vi "DigitalIOWrapper.vi"(0 "error in":errorcluster, 2 "Component IDs":T1[](array[typedef]), 3 "True Only (T)":bool=TRUE) -> (1 "error out":errorcluster, 4 "Changed_IO":T2(array[cluster]))   [LabVIEW 2015]
doc: "Fill the Component IDs array with the full names of digital inputs of interest. Returns the name and digital IO state of any input that has changed since last time.\n\nIf True Only is set, then only returns inputs whose value has changed to true (state != 0)"
uses:
  ROS/Code/SubVIs/DigitalIOComponents.ctl
panel:
  out "changed_io size":i32
  in  "EventWrappers":T2(array[cluster])
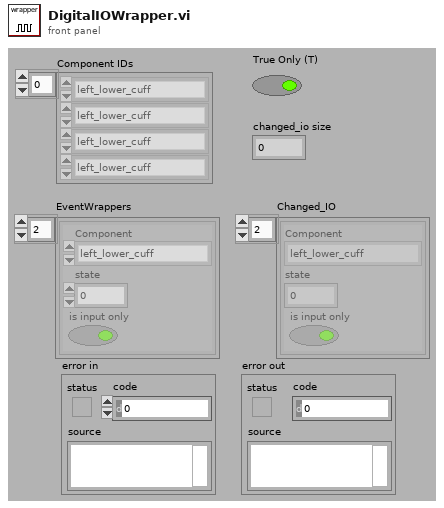
[diagram p1: front panel]
types:
  T1 = typedef "DigitalIOComponents.ctl" = enum16{"left_lower_cuff", "right_lower_cuff", "left_lower_button", "right_lower_button", "left_upper_button", "right_upper_button", "left_shoulder_button", "right_shoulder_button"}
  T2 = cluster{"Component":T1, "state":i8, "is input only":bool}[]
  T3 = cluster{"Component":T1, "state":i8, "is input only":bool}
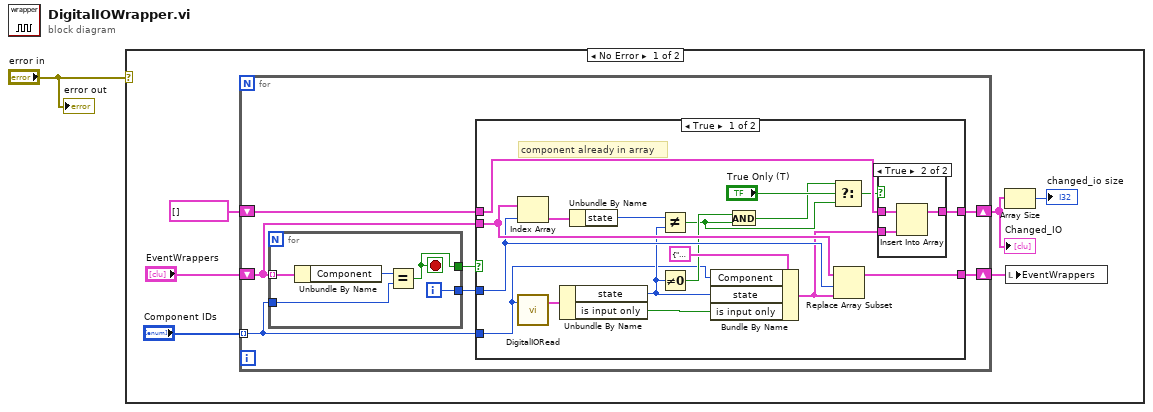
[diagram p0: block diagram]
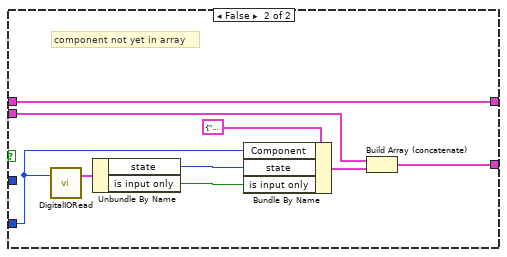
[diagram p3: hidden frame]
diagram:
  n1 = case shown="No Error" "error in" {
    frame No Error {
      n2 = for {
        tunnel: "Component IDs" -> [w8] mode=indexing
        shift-right: [w11] -> w6
        shift-left: "EventWrappers" -> [w12]
        shift-right: [w9] -> w4
        shift-left: T2 [] ("ChangedEvents") -> [w10]
        n3 = for {
          tunnel: w8 -> [w15]
          tunnel: [w16] -> w14
          tunnel: [w19] -> w13
          tunnel: w12 -> [w18] mode=indexing
          i -> [w19]
          stop <- w16 stop-if-true
          n4 = Unbundle By Name(w18) -> ("Component"=w17:T1)
          n5 = Equal?(x=w17, y=w15) -> (x = y?=w16:bool)
        }
        n6 = case shown="True" w14 {
          tunnel: w13 -> [w32 _]
          tunnel: w8 -> [w20 w43]
          tunnel: w12 -> [w33 w50]
          tunnel: [w34 w49] -> w11
          tunnel: w10 -> [w29 w48]
          tunnel: [w27 w48] -> w9
          frame True {
            # "component already in array"
            n7 = Index Array(array=w33, index=w32) -> (element=w31:T3)
            n8 = call "DigitalIORead.vi"("Component"=w20) -> ("Digital IO State"=w36:cluster{"state":i8, "is input only":bool})  [unwired: 2 in, 1 out]
            n9 = Unbundle By Name(w36) -> ("state"=w25:i8, "is input only"=w35:bool)
            n10 = Unbundle By Name(w31) -> ("state"=w30:i8)
            n11 = Not Equal?(x=w30, y=w25) -> (x != y?=w22:bool)
            n12 = Not Equal To 0?(x=w25) -> (x != 0?=w24:bool)
            n13 = Bundle By Name(cluster=T3 {"Component"=enum."right_lower_cuff", "state"=0, "is input only"=TRUE} ("Digital IO Event Wrapper"), "Component"=w20, "state"=w25, "is input only"=w35) -> (w28:T3)
            n14 = And(x=w24, y=w22) -> (x .and. y?=w23:bool)
            n15 = Select(t=w23, s="True Only (T)", f=w22) -> (s? t:f=w21:bool)
            n16 = Replace Array Subset(array=w33, new element=w28, index=w32) -> (w34:T2)
            n17 = case shown="True" w21 {
              tunnel: w29 -> [w38 w41]
              tunnel: w28 -> [_ w40]
              tunnel: [w38 w39] -> w27
              frame False {
              }
              frame True {
                n18 = Insert Into Array(array=w41, new element=w40) -> (w39:T2)  [unwired: 1 in]
              }
            }
          }
          frame False {
            # "component not yet in array"
            n19 = call "DigitalIORead.vi"("Component"=w43) -> ("Digital IO State"=w45:cluster{"state":i8, "is input only":bool})  [unwired: 2 in, 1 out]
            n20 = Unbundle By Name(w45) -> ("state"=w47:i8, "is input only"=w46:bool)
            n21 = Bundle By Name(cluster=T3 {"Component"=enum."right_lower_cuff", "state"=0, "is input only"=TRUE} ("Digital IO Event Wrapper"), "Component"=w43, "state"=w47, "is input only"=w46) -> (w42:T3)
            n22 = Build Array (concatenate)(w50, w42) -> (w49:T2)
          }
        }
      }
      "Changed_IO" <- w4
      n23 = Array Size(array=w4) -> (size(s)=→"changed_io size":i32)
      n24 = local write "EventWrappers"(w6) -> ()
    }
    frame Error {
    }
  }
  "error out" <- "error in"
